vi "Begin.vi"(8 "error in":errorcluster) -> (0 "error out":errorcluster)   [LabVIEW 2015]
doc: "Called before other user functions, this VI is expected to open initial I/O refnums, load in file data, and do all program initialization. Notice that the <B>error out</B> terminal is simply used for data flow. Wiring it to other structures or subVIs ensures that this VI runs first."
uses:
  <vilib>/Rock Robotics/WPI/DriverStation/WPI_DriverStationRobotMode2.ctl
  <vilib>/Rock Robotics/WPI/Joystick/WPI_JoystickDeviceEnum.ctl
  <vilib>/Rock Robotics/WPI/Solenoid/WPI_SolenoidChannel.ctl
  <vilib>/Rock Robotics/SystemInterfaces/DIO/FPGA_DIOPWMChannel.ctl
  <vilib>/Rock Robotics/SystemInterfaces/AI/FPGA_AIChannel.ctl
  <vilib>/Rock Robotics/WPI/SafetyOutput/WPI_SafetyOutputConfigMenu.ctl
  <vilib>/Rock Robotics/SystemInterfaces/DIO/FPGA_DIOChannel.ctl
  <vilib>/Rock Robotics/WPI/Encoder/WPI_EncoderType.ctl
  <vilib>/Rock Robotics/WPI/CAN/TalonSRX/WPI_CANTalonSRX_APIFeedbackSelect.ctl
  <vilib>/Rock Robotics/WPI/CAN/TalonSRX/WPI_CANTalonSRX_APIControlMode.ctl
  <vilib>/Rock Robotics/SystemInterfaces/DIO/FPGA_DIORelayChannel.ctl
  <vilib>/Rock Robotics/SystemInterfaces/spilib/spi_bus.ctl
  Robot Global Data.vi
  <vilib>/Rock Robotics/Network Tables/NT Write String Array.vi
  <vilib>/Rock Robotics/WPI/Solenoid/WPI_SolenoidOpenSingle.vi
  <vilib>/Rock Robotics/WPI/Solenoid/Deprecated/WPI_SolenoidSetBool.vi
  <vilib>/Rock Robotics/WPI/MotorControl/WPI_MotorControlOpen Talon.vi
  <vilib>/Rock Robotics/WPI/RobotDrive/WPI_RobotDriveOpen2MotorWithVictorSP.vi
  <vilib>/Rock Robotics/WPI/Counter/WPI_CounterDigitalInputToDigitalSource.vi
  <vilib>/Rock Robotics/WPI/MotorControl/WPI_MotorControlOpenCANTalonSRX.vi
  <vilib>/Rock Robotics/WPI/MotorControl/WPI_MotorControlOpen VictorSP.vi
  <vilib>/Rock Robotics/WPI/Gyro/WPI_GyroXRS450_SPI_Open.vi
  <vilib>/Rock Robotics/WPI/Switch/WPI_SwitchOpenLimit.vi
  <vilib>/Rock Robotics/WPI/RobotDrive/WPI_RobotDriveOpen4MotorWithVictorSP.vi
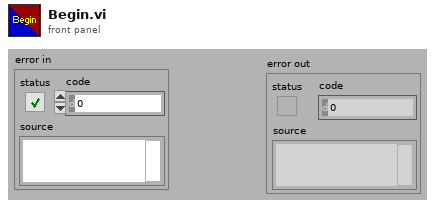
[diagram p1: front panel]
types:
  T1 = typedef "WPI_SolenoidChannel.ctl" = enum8{"Solenoid 0", "Solenoid 1", "Solenoid 2", "Solenoid 3", "Solenoid 4", "Solenoid 5", "Solenoid 6", "Solenoid 7", "Invalid"}
  T2 = typedef "FPGA_DIOPWMChannel.ctl" = enum8{"PWM 0", "PWM 1", "PWM 2", "PWM 3", "PWM 4", "PWM 5", "PWM 6", "PWM 7", "PWM 8", "PWM 9", "PWM MXP 0", "PWM MXP 1", "PWM MXP 2", "PWM MXP 3", "PWM MXP 4", "PWM MXP 5", "PWM MXP 6", "PWM MXP 7", "PWM MXP 8", "PWM MXP 9", "Invalid"}
  T3 = typedef "FPGA_DIOChannel.ctl" = enum8{"DIO 0", "DIO 1", "DIO 2", "DIO 3", "DIO 4", "DIO 5", "DIO 6", "DIO 7", "DIO 8", "DIO 9", "DIO MXP 0", "DIO MXP 1", "DIO MXP 2", "DIO MXP 3", "DIO MXP 4", "DIO MXP 5", "DIO MXP 6", "DIO MXP 7", "DIO MXP 8", "DIO MXP 9", "DIO MXP 10", "DIO MXP 11", "DIO MXP 12", "DIO MXP 13", "DIO MXP 14", "DIO MXP 15", "Invalid"}
  T4 = typedef "spi_bus.ctl" = enum16{"SPI On-Board, CS0", "SPI On-Board, CS1", "SPI On-Board, CS2", "SPI On-Board, CS3", "SPI MXP", "Invalid"}
  T5 = typedef "FPGA_AIChannel.ctl" = enum8{"AI 0", "AI 1", "AI 2", "AI 3", "AI MXP 0", "AI MXP 1", "AI MXP 2", "AI MXP 3", "Invalid"}
  T6 = typedef "FPGA_DIORelayChannel.ctl" = enum8{"Relay 0", "Relay 1", "Relay 2", "Relay 3", "Invalid"}
  T7 = typedef "WPI_CANTalonSRX_APIControlMode.ctl" = enum8{"Percent VBus", "Speed", "Position", "Slave", "Unchanged / Invalid", "Voltage Compensation", "Current", "Motion Profile"}
  T8 = typedef "WPI_CANTalonSRX_APIFeedbackSelect.ctl" = enum16{"Digital Quadrature Encoder", "Analog Potentiometer", "Analog Encoder", "Count on Quad-A (Rising-Edge)", "Count on Quad-A (Falling-Edge)", "CTR Magnetic Enc (Absolute)", "CTR Magnetic Enc (Relative)", "Pulse Width"}
  T9 = typedef "WPI_EncoderType.ctl" = enum16{"1x", "2x", "4x"}
  T10 = typedef "WPI_SafetyOutputConfigMenu.ctl" = enum16{"Enable", "Disable"}
  T11 = enum16{"Intake", "Fender", "D4", "Low Bar", "Backwards Fender"}
  T12 = typedef "WPI_JoystickDeviceEnum.ctl" = enum16{"USB 0", "USB 1", "USB 2", "USB 3", "USB 4", "USB 5"}
  T13 = typedef "WPI_DriverStationRobotMode2.ctl" = enum16{"Autonomous Disabled", "Autonomous Enabled", "Teleop Disabled", "Teleop Enabled", "Disconnected", "Finish", "Test Disabled", "Test Enabled", "Emergency Stopped"}
  T14 = typedef "WPI_MotorControlDeviceRef.ctl" = cluster{"DeviceStatus":errorcluster, "Type":T15, "PWM":cluster{"PWM Channel":T2, "DeadBand":T16}, "CAN":cluster{"Device Number":u8, "Control Mode":T17, "Semaphore":T18, "Max Vout":dbl, "TalonSRX Control Mode":T7}, "Invert":bool}
  T15 = typedef "WPI_MotorControlType.ctl" = enum16{"PWM", "CAN", "CANTalonSRX"}
  T16 = typedef "WPI_PWMDeadband.ctl" = cluster{"Name":string, "maxPositivePwm":i32, "minPositivePwm":i32, "centerPwm":i32, "maxNegativePwm":i32, "minNegativePwm":i32, "angularRange":u16}
  T17 = typedef "WPI_CANJaguar_ControlMode.ctl" = enum8{"Percent VBus", "Current", "Speed", "Position", "Voltage"}
  T18 = typedef "Semaphore RefNum" = refnum<k1>
  T19 = typedef "WPI_RobotDriveDevRef.ctl" = cluster{"DevStatus":errorcluster, "Motors[]":T14[], "Square Inputs":bool, "Max Output":dbl}
  T20 = typedef "WPI_RelayDevRef.ctl" = cluster{"DevStatus":errorcluster, "Relay Channel":T6, "Relay Direction":T21}
  T21 = typedef "WPI_RelayDirection.ctl" = enum16{"Both directions", "Forward only", "Reverse only"}
  T22 = typedef "WPI_SolenoidDevRef.ctl" = cluster{"DevStatus":errorcluster, "Pneumatics Control Module":u8, "Forward Solenoid Channel":T1, "Reverse Solenoid Channel":T1}
  T23 = typedef "WPI_GyroDevRef.ctl" = cluster{"DevStatus":errorcluster, "Analog Channel":T5, "Offset":dbl, "Gain (VoltsPerDegree/Second)":dbl, "Gyro Type":enum16{"Analog", "XRS450"}, "Handle":i32, "SPI Bus":T4, "Device Found":bool, "Sample Rate":dbl, "Calibrate On Open":bool}
  T24 = typedef "WPI_PotentiometerDevRef.ctl" = cluster{"DevStatus":errorcluster, "Analog Channel":T5, "Invert Output":bool}
  T25 = typedef "WPI_JoystickDevRef.ctl" = cluster{"Device":T12}
  T26 = typedef "WPI_SwitchDevRef.ctl" = cluster{"DevStatus":errorcluster, "DIO Channel":T3, "CntIndex":T27, "Normally Closed":bool}
  T27 = typedef "FPGA_CounterCtrSystemIndex.ctl" = enum8{"Ctr 0", "Ctr 1", "Ctr 2", "Ctr 3", "Ctr 4", "Ctr 5", "Ctr 6", "Ctr 7", "Invalid"}
  T28 = typedef "WPI_DigitalInputDevRef.ctl" = cluster{"DevStatus":errorcluster, "DIO Channel":T3}
  T29 = typedef "FPGA_CounterEncoderSourceConvertionLVSourceType.ctl" = cluster{"DevStatus":errorcluster, "AnalogTriggerMode?":bool, "DigitalMode":cluster{"DIO Channel":T30}, "AnalogTriggerMode":cluster{"AnalogTriggerIndex":T31, "OutputType":T32}}
  T30 = typedef "FPGA_DIODigitalSourceChannel.ctl" = enum8{"DIO 0", "DIO 1", "DIO 2", "DIO 3", "DIO 4", "DIO 5", "DIO 6", "DIO 7", "DIO 8", "DIO 9", "DIO MXP 0", "DIO MXP 1", "DIO MXP 2", "DIO MXP 3", "DIO MXP 4", "DIO MXP 5", "DIO MXP 6", "DIO MXP 7", "DIO MXP 8", "DIO MXP 9", "DIO MXP 10", "DIO MXP 11", "DIO MXP 12", "DIO MXP 13", "DIO MXP 14", "DIO MXP 15", "Disabled"}
  T31 = typedef "FPGA_AnalogTriggerIndex.ctl" = enum8{"Trig 0", "Trig 1", "Trig 2", "Trig 3", "Trig 4", "Trig 5", "Trig 6", "Trig 7", "Invalid"}
  T32 = typedef "FPGA_AnalogTriggerOutType.ctl" = enum16{"InWindow", "TriggerState", "Rising", "Falling"}
  T33 = typedef "WPI_AnalogChannelDevRef.ctl" = cluster{"DevStatus":errorcluster, "Analog Channel":T5}
  T34 = typedef "WPI_EncoderDevRef.ctl" = cluster{"DevStatus":errorcluster, "EncoderIndex":T35, "CounterIndex":T27, "DistancePerCount":dbl, "Decoding Type":T9}
  T35 = typedef "FPGA_EncoderIdx.ctl" = enum8{"Enc 0", "Enc 1", "Enc 2", "Enc 3", "Enc 4", "Enc 5", "Enc 6", "Enc 7", "Invalid"}
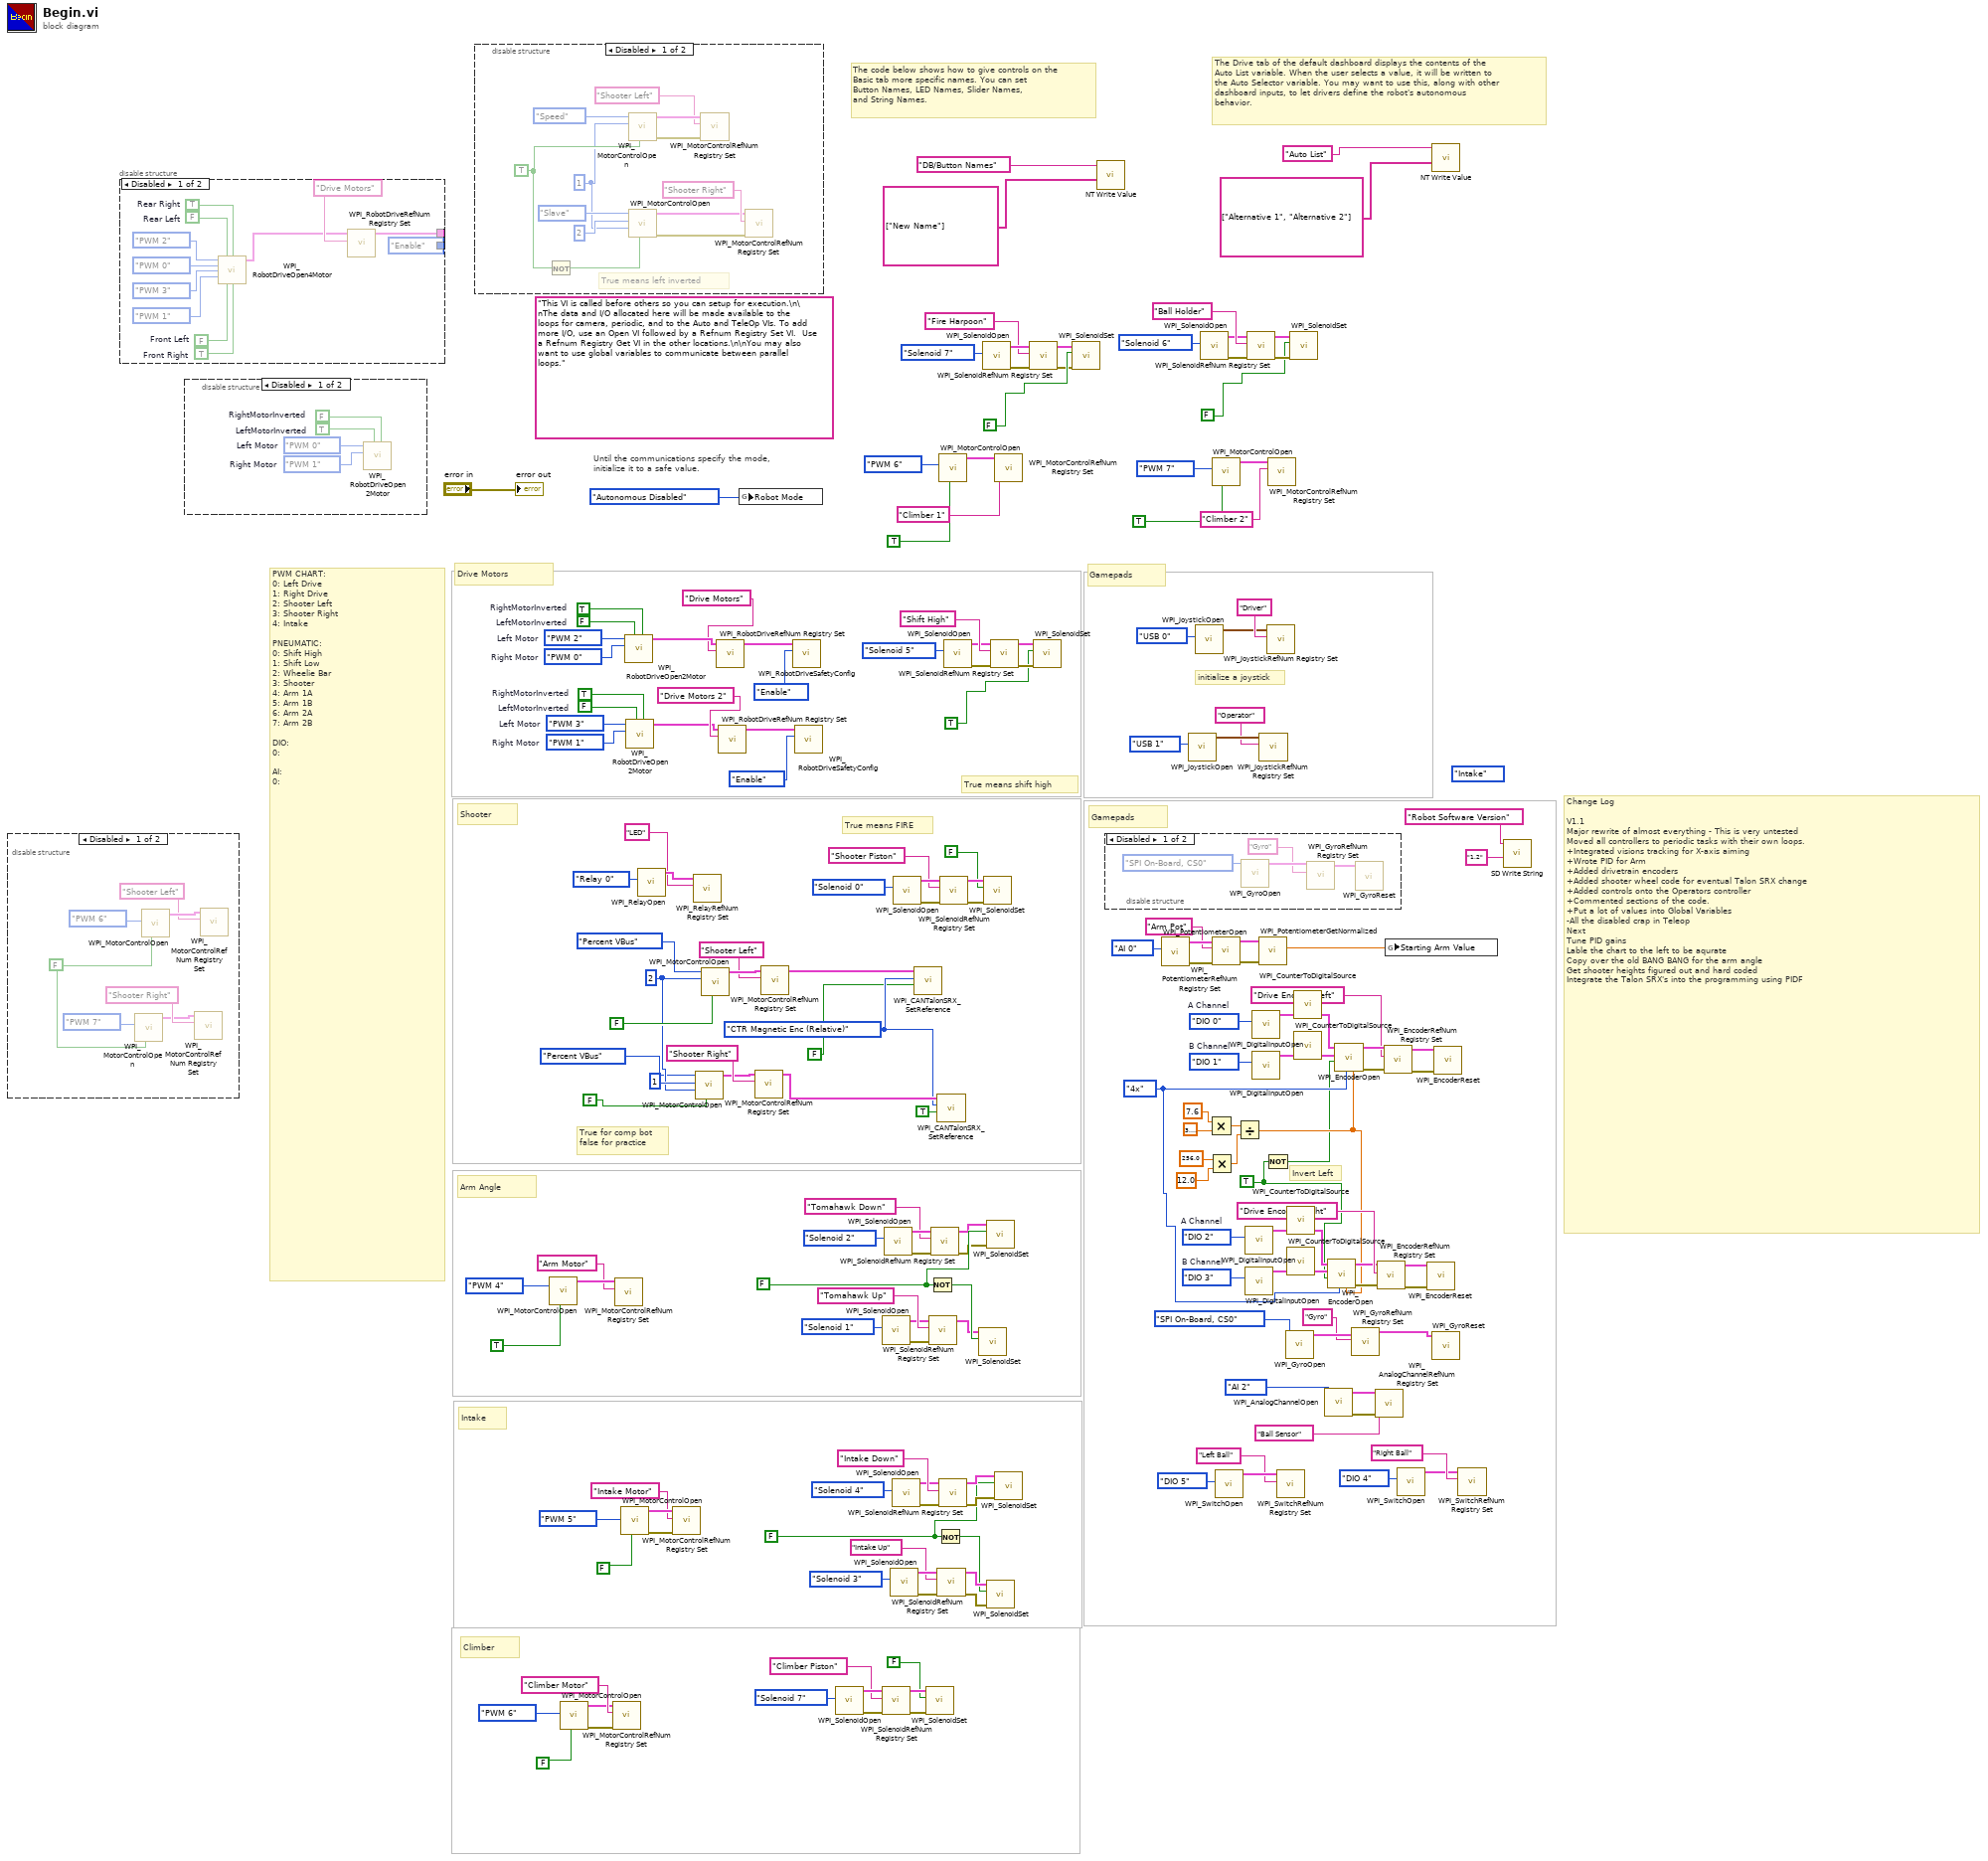
[diagram p0: block diagram]
diagram:
  w70 = FALSE
  w53 = WPI_CANTalonSRX_APIFeedbackSelect."CTR Magnetic Enc (Relative)" ("Feedback Reference")
  w75 = u8 2 ("Device Number")
  w84 = TRUE
  w88 = FPGA_DIOChannel."DIO 3"  # B Channel
  w89 = FPGA_DIOChannel."DIO 2"  # A Channel
  w87 = WPI_EncoderType."4x" ("Decoding Type")
  w114 = FPGA_DIOChannel."DIO 1"  # B Channel
  w113 = FPGA_DIOChannel."DIO 0"  # A Channel
  w117 = FPGA_DIOPWMChannel."PWM 1"  # Right Motor
  w118 = FPGA_DIOPWMChannel."PWM 3"  # Left Motor
  w119 = FALSE  # LeftMotorInverted
  w120 = TRUE  # RightMotorInverted
  w132 = FPGA_DIOPWMChannel."PWM 0"  # Right Motor
  w131 = FPGA_DIOPWMChannel."PWM 2"  # Left Motor
  w130 = FALSE  # LeftMotorInverted
  w129 = TRUE  # RightMotorInverted
  (unwired) T11."Intake"
  w153 = FALSE
  (unwired) "This VI is called before others so you can setup for execution.\n\nThe data and I/O allocated here will be made available to the loops for camera, periodic, and to the Auto and TeleOp VIs. To add more I/O, use an Open VI followed by a Refnum Registry Set VI.  Use a Refnum Registry Get VI in the other locations.\n\nYou may also want to use global variables to communicate between parallel loops."
  # "Climber"
  # "True for comp bot\nfalse for practice"
  # "Change Log\n \nV1.1\nMajor rewrite of almost everything - This is very untested\nMoved all controllers to periodic tasks with their own loops.\n+Integrated visions tracking for X-axis aiming\n+Wrote PID for Arm\n+Added drivetrain encoders\n+Added shooter wheel code for eventual Talon SRX change\n+Added controls onto the Operators controller \n+Commented sections of the code.\n+Put a lot of values into Global Variables\n-All the disabled crap in Teleop\nNext\nTune PID gains\nLable the chart to the left to be aqurate\nCopy over the old BANG BANG for the arm angle\nGet shooter heights figured out and hard coded\nIntegrate the Talon SRX's into the programming using PIDF"
  # "Invert Left"
  # "Gamepads"
  # "True means FIRE"
  # "True means shift high"
  # "Intake"
  # "Arm Angle"
  # "Shooter"
  # "Gamepads"
  # "Drive Motors"
  # "PWM CHART:\n0: Left Drive\n1: Right Drive\n2: Shooter Left\n3: Shooter Right\n4: Intake \n\nPNEUMATIC:\n0: Shift High\n1: Shift Low\n2: Wheelie Bar\n3: Shooter \n4: Arm 1A\n5: Arm 1B\n6: Arm 2A\n7: Arm 2B \n\nDIO:\n0: \n\nAI:\n0:"
  # "The Drive tab of the default dashboard displays the contents of the\nAuto List variable. When the user selects a value, it will be written to\nthe Auto Selector variable. You may want to use this, along with other\ndashboard inputs, to let drivers define the robot's autonomous\nbehavior."
  # "The code below shows how to give controls on the\nBasic tab more specific names. You can set\nButton Names, LED Names, Slider Names,\nand String Names."
  # "initialize a joystick"
  # "Until the communications specify the mode,\ninitialize it to a safe value."
  n1 = disable-structure shown="Disabled" {
    frame Disabled {
      w186 = FALSE
      n2 = call-poly <vilib>:"WPI_MotorControlOpen.vi"("Invert"=w186, "PWM Channel"=FPGA_DIOPWMChannel."PWM 7") -> ("MotorControlDeviceRef"=w188:T14)  [unwired: 8 in, 1 out]
      n3 = call-poly <vilib>:"WPI_MotorControlOpen.vi"("Invert"=w186, "PWM Channel"=FPGA_DIOPWMChannel."PWM 6") -> ("MotorControlDeviceRef"=w191:T14)  [unwired: 8 in, 1 out]
      n4 = call <vilib>:"WPI_MotorControlRefNum Registry Set.vi"("refnum name"="Shooter Right", "MotorControlDevRef"=w188) -> ()  [unwired: 8 in, 2 out]
      n5 = call <vilib>:"WPI_MotorControlRefNum Registry Set.vi"("refnum name"="Shooter Left", "MotorControlDevRef"=w191) -> ()  [unwired: 8 in, 2 out]
    }
    frame Enabled {
    }
  }
  n6 = disable-structure shown="Disabled" {
    disable-tunnel: [w203 _] -> _
    disable-tunnel: [WPI_SafetyOutputConfigMenu."Enable" ("mode") _] -> _
    frame Disabled {
      w195 = FALSE  # Rear Left
      w194 = TRUE  # Rear Right
      w196 = TRUE  # Front Right
      w197 = FALSE  # Front Left
      n7 = call-poly <vilib>:"WPI_RobotDriveOpen4Motor.vi"("Rear Left Motor"=FPGA_DIOPWMChannel."PWM 2", "Rear Left Motor Inverted"=w195, "Rear Right Motor Inverted"=w194, "Rear Right Motor"=FPGA_DIOPWMChannel."PWM 0", "Front Left Motor"=FPGA_DIOPWMChannel."PWM 3", "Front Right Motor"=FPGA_DIOPWMChannel."PWM 1", "Front Left Motor Inverted"=w197, "Front Right Motor Inverted"=w196) -> ("RobotDriveDevRef"=w193:T19)  [unwired: 6 in, 1 out]
      n8 = call <vilib>:"WPI_RobotDriveRefNum Registry Set.vi"("refnum name"="Drive Motors", "RobotDriveDevRef"=w193) -> ("RobotDriveDevRef"=w203:T19)  [unwired: 2 in, 7 out]
    }
    frame Enabled {
    }
  }
  n9 = disable-structure shown="Disabled" {
    frame Disabled {
      w205 = FPGA_DIOPWMChannel."PWM 1"  # Right Motor
      w206 = FPGA_DIOPWMChannel."PWM 0"  # Left Motor
      w207 = TRUE  # LeftMotorInverted
      w208 = FALSE  # RightMotorInverted
      n10 = call-poly <vilib>:"WPI_RobotDriveOpen2Motor.vi"("Right Motor Inverted"=w208, "Left Motor Inverted"=w207, "Right Motor"=w205, "Left Motor"=w206) -> ()  [unwired: 1 in, 7 out]
    }
    frame Enabled {
    }
  }
  n11 = disable-structure shown="Disabled" {
    frame Disabled {
      w209 = u8 1 ("Device Number")
      w213 = TRUE
      # "True means left inverted"
      n12 = Not(x=w213) -> (.not. x?=w214:bool)
      n13 = call-poly <vilib>:"WPI_MotorControlOpen.vi"("Invert"=w213, "Device Number"=w209, "Control Mode"=WPI_CANTalonSRX_APIControlMode."Speed") -> ("error out"=w220:errorcluster, "MotorControlDeviceRef"=w219:T14)  [unwired: 7 in]
      n14 = call-poly <vilib>:"WPI_MotorControlOpen.vi"("Invert"=w214, "Master Device Number"=w209, "Device Number"=u8 2, "Control Mode"=WPI_CANTalonSRX_APIControlMode."Slave") -> ("error out"=w215:errorcluster, "MotorControlDeviceRef"=w216:T14)  [unwired: 6 in]
      n15 = call <vilib>:"WPI_MotorControlRefNum Registry Set.vi"("error in (no error)"=w220, "refnum name"="Shooter Left", "MotorControlDevRef"=w219) -> ()  [unwired: 7 in, 2 out]
      n16 = call <vilib>:"WPI_MotorControlRefNum Registry Set.vi"("error in (no error)"=w215, "refnum name"="Shooter Right", "MotorControlDevRef"=w216) -> ()  [unwired: 7 in, 2 out]
    }
    frame Enabled {
    }
  }
  n17 = call-poly <vilib>:"WPI_MotorControlOpen.vi"("Invert"=TRUE, "PWM Channel"=FPGA_DIOPWMChannel."PWM 4") -> ("MotorControlDeviceRef"=w141:T14)  [unwired: 8 in, 1 out]
  n18 = call-poly <vilib>:"WPI_MotorControlOpen.vi"("Invert"=FALSE, "PWM Channel"=FPGA_DIOPWMChannel."PWM 6") -> ("error out"=w8:errorcluster, "MotorControlDeviceRef"=w9:T14)  [unwired: 8 in]
  n19 = call <vilib>:"WPI_MotorControlRefNum Registry Set.vi"("error in (no error)"=w8, "refnum name"="Climber Motor", "MotorControlDevRef"=w9) -> ()  [unwired: 7 in, 2 out]
  n20 = call <vilib>:"WPI_MotorControlRefNum Registry Set.vi"("refnum name"="Arm Motor", "MotorControlDevRef"=w141) -> ()  [unwired: 8 in, 2 out]
  n21 = call-poly <vilib>:"WPI_MotorControlOpen.vi"("Invert"=FALSE, "PWM Channel"=FPGA_DIOPWMChannel."PWM 5") -> ("error out"=w152:errorcluster, "MotorControlDeviceRef"=w151:T14)  [unwired: 8 in]
  n22 = call-poly <vilib>:"WPI_RobotDriveOpen2Motor.vi"("Right Motor Inverted"=w129, "Left Motor Inverted"=w130, "Right Motor"=w132, "Left Motor"=w131) -> ("RobotDriveDevRef"=w128:T19)  [unwired: 1 in, 6 out]
  n23 = call-poly <vilib>:"WPI_RobotDriveOpen2Motor.vi"("Right Motor Inverted"=w120, "Left Motor Inverted"=w119, "Right Motor"=w117, "Left Motor"=w118) -> ("RobotDriveDevRef"=w121:T19)  [unwired: 1 in, 6 out]
  n24 = call <vilib>:"WPI_RelayOpen.vi"("Relay Channel"=FPGA_DIORelayChannel."Relay 0") -> ("RelayDevRef"=w57:T20)  [unwired: 9 in, 1 out]
  n25 = call <vilib>:"WPI_MotorControlRefNum Registry Set.vi"("error in (no error)"=w152, "refnum name"="Intake Motor", "MotorControlDevRef"=w151) -> ()  [unwired: 7 in, 2 out]
  n26 = call <vilib>:"WPI_RelayRefNum Registry Set.vi"("refnum name"="LED", "RelayDevRef"=w57) -> ()  [unwired: 8 in, 2 out]
  n27 = call-poly <vilib>:"WPI_MotorControlOpen.vi"("Invert"=FALSE, "Master Device Number"=w75, "Device Number"=u8 1, "Control Mode"=WPI_CANTalonSRX_APIControlMode."Percent VBus") -> ("MotorControlDeviceRef"=w78:T14)  [unwired: 6 in, 1 out]
  n28 = call-poly <vilib>:"WPI_MotorControlOpen.vi"("Invert"=FALSE, "Device Number"=w75, "Control Mode"=WPI_CANTalonSRX_APIControlMode."Percent VBus") -> ("MotorControlDeviceRef"=w81:T14)  [unwired: 7 in, 1 out]
  n29 = call <vilib>:"WPI_RobotDriveRefNum Registry Set.vi"("refnum name"="Drive Motors", "RobotDriveDevRef"=w128) -> ("RobotDriveDevRef"=w127:T19)  [unwired: 2 in, 7 out]
  n30 = call <vilib>:"WPI_RobotDriveRefNum Registry Set.vi"("refnum name"="Drive Motors 2", "RobotDriveDevRef"=w121) -> ("RobotDriveDevRef"=w122:T19)  [unwired: 2 in, 7 out]
  n31 = global write "Robot Global Data.vi" "Robot Mode"(WPI_DriverStationRobotMode2."Autonomous Disabled" ("Robot Mode")) -> ()
  n32 = call <vilib>:"WPI_MotorControlRefNum Registry Set.vi"("refnum name"="Shooter Right", "MotorControlDevRef"=w78) -> ("MotorControlDevRef"=w54:T14)  [unwired: 8 in, 1 out]
  n33 = call <vilib>:"WPI_MotorControlRefNum Registry Set.vi"("refnum name"="Shooter Left", "MotorControlDevRef"=w81) -> ("MotorControlDevRef"=w73:T14)  [unwired: 8 in, 1 out]
  n34 = call <vilib>:"WPI_RobotDriveSafetyConfig.vi"("mode"=WPI_SafetyOutputConfigMenu."Enable", "RobotDriveDevRef"=w127) -> ()  [unwired: 8 in, 2 out]
  n35 = call <vilib>:"WPI_RobotDriveSafetyConfig.vi"("mode"=WPI_SafetyOutputConfigMenu."Enable", "RobotDriveDevRef"=w122) -> ()  [unwired: 8 in, 2 out]
  n36 = call-poly <vilib>:"WPI_SolenoidOpen.vi"("Solenoid Channel"=WPI_SolenoidChannel."Solenoid 7") -> ("error out"=w7:errorcluster, "SolenoidDevRef"=w6:T22)  [unwired: 9 in]
  n37 = call-poly <vilib>:"WPI_SolenoidOpen.vi"("Solenoid Channel"=WPI_SolenoidChannel."Solenoid 1") -> ("error out"=w62:errorcluster, "SolenoidDevRef"=w63:T22)  [unwired: 9 in]
  n38 = call <vilib>:"WPI_SolenoidRefNum Registry Set.vi"("error in (no error)"=w7, "refnum name"="Climber Piston", "SolenoidDevRef"=w6) -> ("error out"=w3:errorcluster, "SolenoidDevRef"=w2:T22)  [unwired: 7 in]
  n39 = call-poly <vilib>:"WPI_SolenoidOpen.vi"("Solenoid Channel"=WPI_SolenoidChannel."Solenoid 2") -> ("error out"=w61:errorcluster, "SolenoidDevRef"=w60:T22)  [unwired: 9 in]
  n40 = call-poly <vilib>:"WPI_SolenoidOpen.vi"("Solenoid Channel"=WPI_SolenoidChannel."Solenoid 3") -> ("error out"=w162:errorcluster, "SolenoidDevRef"=w161:T22)  [unwired: 9 in]
  n41 = call-poly <vilib>:"WPI_SolenoidOpen.vi"("Solenoid Channel"=WPI_SolenoidChannel."Solenoid 4") -> ("error out"=w163:errorcluster, "SolenoidDevRef"=w164:T22)  [unwired: 9 in]
  n42 = call-poly <vilib>:"WPI_SolenoidOpen.vi"("Solenoid Channel"=WPI_SolenoidChannel."Solenoid 0") -> ("error out"=w173:errorcluster, "SolenoidDevRef"=w172:T22)  [unwired: 9 in]
  n43 = call <vilib>:"WPI_CANTalonSRX_SetReference.vi"("Reverse Feedback Sensor"=FALSE, "Feedback Reference"=w53, "CAN Talon SRX Ref"=w73) -> ()  [unwired: 7 in, 2 out]
  n44 = call-poly <vilib>:"WPI_SolenoidSet.vi"("error in (no error)"=w3, "Value"=FALSE, "SolenoidDevRef"=w2) -> ()  [unwired: 7 in, 2 out]
  n45 = Not(x=w70) -> (.not. x?=w69:bool)
  n46 = call <vilib>:"WPI_SolenoidRefNum Registry Set.vi"("error in (no error)"=w62, "refnum name"="Tomahawk Up", "SolenoidDevRef"=w63) -> ("SolenoidDevRef"=w66:T22)  [unwired: 7 in, 1 out]
  n47 = call <vilib>:"WPI_SolenoidRefNum Registry Set.vi"("error in (no error)"=w61, "refnum name"="Tomahawk Down", "SolenoidDevRef"=w60) -> ("error out"=w67:errorcluster, "SolenoidDevRef"=w68:T22)  [unwired: 7 in]
  n48 = Not(x=w153) -> (.not. x?=w154:bool)
  n49 = call <vilib>:"WPI_CANTalonSRX_SetReference.vi"("Reverse Feedback Sensor"=TRUE, "Feedback Reference"=w53, "CAN Talon SRX Ref"=w54) -> ()  [unwired: 7 in, 2 out]
  n50 = call <vilib>:"WPI_SolenoidRefNum Registry Set.vi"("error in (no error)"=w162, "refnum name"="Intake Up", "SolenoidDevRef"=w161) -> ("error out"=w158:errorcluster, "SolenoidDevRef"=w157:T22)  [unwired: 7 in]
  n51 = call-poly <vilib>:"WPI_MotorControlOpen.vi"("Invert"=TRUE, "PWM Channel"=FPGA_DIOPWMChannel."PWM 6") -> ("MotorControlDeviceRef"=w28:T14)  [unwired: 8 in, 1 out]
  n52 = call <vilib>:"WPI_SolenoidRefNum Registry Set.vi"("error in (no error)"=w163, "refnum name"="Intake Down", "SolenoidDevRef"=w164) -> ("error out"=w156:errorcluster, "SolenoidDevRef"=w155:T22)  [unwired: 7 in]
  n53 = call <vilib>:"WPI_SolenoidRefNum Registry Set.vi"("error in (no error)"=w173, "refnum name"="Shooter Piston", "SolenoidDevRef"=w172) -> ("error out"=w169:errorcluster, "SolenoidDevRef"=w168:T22)  [unwired: 7 in]
  n54 = call-poly <vilib>:"WPI_SolenoidOpen.vi"("Solenoid Channel"=WPI_SolenoidChannel."Solenoid 5") -> ("error out"=w144:errorcluster, "SolenoidDevRef"=w145:T22)  [unwired: 9 in]
  n55 = call-poly <vilib>:"WPI_SolenoidSet.vi"("Value"=w69, "SolenoidDevRef"=w66) -> ()  [unwired: 8 in, 2 out]
  n56 = call-poly <vilib>:"WPI_SolenoidOpen.vi"("Solenoid Channel"=WPI_SolenoidChannel."Solenoid 7") -> ("error out"=w39:errorcluster, "SolenoidDevRef"=w38:T22)  [unwired: 9 in]
  n57 = call-poly <vilib>:"WPI_SolenoidSet.vi"("error in (no error)"=w169, "Value"=FALSE, "SolenoidDevRef"=w168) -> ()  [unwired: 7 in, 2 out]
  n58 = call-poly <vilib>:"WPI_SolenoidSet.vi"("error in (no error)"=w67, "Value"=w70, "SolenoidDevRef"=w68) -> ()  [unwired: 7 in, 2 out]
  n59 = call-poly <vilib>:"WPI_SolenoidSet.vi"("error in (no error)"=w158, "Value"=w154, "SolenoidDevRef"=w157) -> ()  [unwired: 7 in, 2 out]
  n60 = call <vilib>:"WPI_SolenoidRefNum Registry Set.vi"("error in (no error)"=w144, "refnum name"="Shift High", "SolenoidDevRef"=w145) -> ("error out"=w143:errorcluster, "SolenoidDevRef"=w142:T22)  [unwired: 7 in]
  n61 = call <vilib>:"WPI_MotorControlRefNum Registry Set.vi"("refnum name"="Climber 1", "MotorControlDevRef"=w28) -> ()  [unwired: 8 in, 2 out]
  n62 = call-poly <vilib>:"WPI_SolenoidSet.vi"("error in (no error)"=w156, "Value"=w153, "SolenoidDevRef"=w155) -> ()  [unwired: 7 in, 2 out]
  n63 = call <vilib>:"WPI_SolenoidRefNum Registry Set.vi"("error in (no error)"=w39, "refnum name"="Fire Harpoon", "SolenoidDevRef"=w38) -> ("error out"=w40:errorcluster, "SolenoidDevRef"=w41:T22)  [unwired: 7 in]
  n64 = call-poly <vilib>:"WPI_SolenoidSet.vi"("error in (no error)"=w143, "Value"=TRUE, "SolenoidDevRef"=w142) -> ()  [unwired: 7 in, 2 out]
  n65 = call-poly <vilib>:"WPI_SolenoidSet.vi"("error in (no error)"=w40, "Value"=FALSE, "SolenoidDevRef"=w41) -> ()  [unwired: 7 in, 2 out]
  n66 = call-poly <vilib>:"NT Write Value.vi"("String Array"=string[] ["New Name"], "Name"="DB/Button Names") -> ()  [unwired: 9 in, 1 out]
  n67 = disable-structure shown="Disabled" {
    frame Disabled {
      n68 = call-poly <vilib>:"WPI_GyroOpen.vi"("SPI Bus"=spi_bus."SPI On-Board, CS0") -> ("GyroDevRef"=w224:T23)  [unwired: 9 in, 1 out]
      n69 = call <vilib>:"WPI_GyroRefNum Registry Set.vi"("refnum name"="Gyro", "GyroDevRef"=w224) -> ("GyroDevRef"=w223:T23)  [unwired: 8 in, 1 out]
      n70 = call <vilib>:"WPI_GyroReset.vi"("GyroDevRef"=w223) -> ()  [unwired: 9 in, 2 out]
    }
    frame Enabled {
    }
  }
  n71 = call <vilib>:"WPI_PotentiometerOpen.vi"("Analog Channel"=FPGA_AIChannel."AI 0") -> ("error out"=w139:errorcluster, "PotDevRef"=w138:T24)  [unwired: 9 in]
  n72 = call <vilib>:"WPI_JoystickOpen.vi"("JoystickDevice"=WPI_JoystickDeviceEnum."USB 1") -> ("JoystickDevRef"=w175:T25)  [unwired: 10 in]
  n73 = call <vilib>:"WPI_JoystickOpen.vi"("JoystickDevice"=WPI_JoystickDeviceEnum."USB 0") -> ("JoystickDevRef"=w183:T25)  [unwired: 10 in]
  n74 = call-poly <vilib>:"WPI_SolenoidOpen.vi"("Solenoid Channel"=WPI_SolenoidChannel."Solenoid 6") -> ("error out"=w32:errorcluster, "SolenoidDevRef"=w33:T22)  [unwired: 9 in]
  n75 = Multiply(x=7.6, y=3.141592653589793) -> (x*y=w99:dbl)
  n76 = Multiply(x=256.0, y=12.0) -> (x*y=w102:dbl)
  n77 = call-poly <vilib>:"WPI_MotorControlOpen.vi"("Invert"=TRUE, "PWM Channel"=FPGA_DIOPWMChannel."PWM 7") -> ("MotorControlDeviceRef"=w25:T14)  [unwired: 8 in, 1 out]
  n78 = call <vilib>:"WPI_PotentiometerRefNum Registry Set.vi"("error in (no error)"=w139, "refnum name"="Arm Pot", "PotDevRef"=w138) -> ("error out"=w135:errorcluster, "PotDevRef"=w134:T24)  [unwired: 7 in]
  n79 = call-poly <vilib>:"WPI_SwitchOpen.vi"("DIO Channel"=FPGA_DIOChannel."DIO 5") -> ("SwitchDevRef"=w19:T26)  [unwired: 9 in, 1 out]
  n80 = Divide(x=w99, y=w102) -> (x/y=w86:dbl)
  n81 = call <vilib>:"WPI_DigitalInputOpen.vi"("DIO Channel"=w89) -> ("DigitalInputDevRef"=w92:T28)  [unwired: 1 in, 9 out]
  n82 = call <vilib>:"WPI_DigitalInputOpen.vi"("DIO Channel"=w88) -> ("DigitalInputDevRef"=w91:T28)  [unwired: 1 in, 9 out]
  n83 = call <vilib>:"WPI_SolenoidRefNum Registry Set.vi"("error in (no error)"=w32, "refnum name"="Ball Holder", "SolenoidDevRef"=w33) -> ("error out"=w31:errorcluster, "SolenoidDevRef"=w30:T22)  [unwired: 7 in]
  n84 = call <vilib>:"WPI_DigitalInputOpen.vi"("DIO Channel"=w113) -> ("DigitalInputDevRef"=w110:T28)  [unwired: 1 in, 9 out]
  n85 = call <vilib>:"WPI_DigitalInputOpen.vi"("DIO Channel"=w114) -> ("DigitalInputDevRef"=w111:T28)  [unwired: 1 in, 9 out]
  n86 = call <vilib>:"WPI_PotentiometerGetNormalized.vi"("error in"=w135, "PotDevRef"=w134) -> ("Normalized Value"=w133:dbl)  [unwired: 7 in, 2 out]
  n87 = call <vilib>:"WPI_JoystickRefNum Registry Set.vi"("refnum name"="Operator", "JoystickDevRef"=w175) -> ()  [unwired: 8 in, 2 out]
  n88 = Not(x=w84) -> (.not. x?=w85:bool)
  n89 = call <vilib>:"WPI_JoystickRefNum Registry Set.vi"("refnum name"="Driver", "JoystickDevRef"=w183) -> ()  [unwired: 8 in, 2 out]
  n90 = call <vilib>:"WPI_MotorControlRefNum Registry Set.vi"("refnum name"="Climber 2", "MotorControlDevRef"=w25) -> ()  [unwired: 8 in, 2 out]
  n91 = call <vilib>:"WPI_SwitchRefNum Registry Set.vi"("refnum name"="Left Ball", "SwitchDevRef"=w19) -> ()  [unwired: 8 in, 2 out]
  n92 = call-poly <vilib>:"WPI_GyroOpen.vi"("SPI Bus"=spi_bus."SPI On-Board, CS0") -> ("GyroDevRef"=w50:T23)  [unwired: 9 in, 1 out]
  n93 = call-poly <vilib>:"WPI_CounterToDigitalSource.vi"("DigitalInputDevRef"=w92) -> ("Digital Source"=w93:T29)  [unwired: 6 out]
  n94 = call-poly <vilib>:"WPI_CounterToDigitalSource.vi"("DigitalInputDevRef"=w91) -> ("Digital Source"=w90:T29)  [unwired: 6 out]
  n95 = call-poly <vilib>:"WPI_SolenoidSet.vi"("error in (no error)"=w31, "Value"=FALSE, "SolenoidDevRef"=w30) -> ()  [unwired: 7 in, 2 out]
  n96 = call-poly <vilib>:"WPI_CounterToDigitalSource.vi"("DigitalInputDevRef"=w110) -> ("Digital Source"=w109:T29)  [unwired: 6 out]
  n97 = call-poly <vilib>:"WPI_CounterToDigitalSource.vi"("DigitalInputDevRef"=w111) -> ("Digital Source"=w112:T29)  [unwired: 6 out]
  n98 = call <vilib>:"WPI_AnalogChannelOpen.vi"("Analog Channel"=FPGA_AIChannel."AI 2") -> ("error out"=w46:errorcluster, "AIDeviceRef"=w45:T33)  [unwired: 9 in]
  n99 = call <vilib>:"WPI_EncoderOpen.vi"("DistancePerCount"=w86, "Decoding Type"=w87, "Invert Direction (False)"=w84, "BSource"=w90, "ASource"=w93) -> ("error out"=w94:errorcluster, "EncoderDevRef"=w95:T34)  [unwired: 3 in, 2 out]
  n100 = call <vilib>:"WPI_EncoderOpen.vi"("DistancePerCount"=w86, "Decoding Type"=w87, "Invert Direction (False)"=w85, "BSource"=w112, "ASource"=w109) -> ("error out"=w108:errorcluster, "EncoderDevRef"=w107:T34)  [unwired: 3 in, 2 out]
  n101 = call <vilib>:"WPI_GyroRefNum Registry Set.vi"("refnum name"="Gyro", "GyroDevRef"=w50) -> ("GyroDevRef"=w49:T23)  [unwired: 8 in, 1 out]
  n102 = call <vilib>:"WPI_AnalogChannelRefNum Registry Set.vi"("error in (no error)"=w46, "refnum name"="Ball Sensor", "AIDeviceRef"=w45) -> ()  [unwired: 7 in, 2 out]
  n103 = call <vilib>:"WPI_EncoderRefNum Registry Set.vi"("error in (no error)"=w94, "refnum name"="Drive Encoder Right", "EncoderDevRef"=w95) -> ("error out"=w96:errorcluster, "EncoderDevRef"=w97:T34)  [unwired: 7 in]
  n104 = call <vilib>:"WPI_EncoderRefNum Registry Set.vi"("error in (no error)"=w108, "refnum name"="Drive Encoder Left", "EncoderDevRef"=w107) -> ("error out"=w106:errorcluster, "EncoderDevRef"=w105:T34)  [unwired: 7 in]
  n105 = global write "Robot Global Data.vi" "Starting Arm Value"(w133) -> ()
  n106 = call-poly <vilib>:"WPI_SwitchOpen.vi"("DIO Channel"=FPGA_DIOChannel."DIO 4") -> ("SwitchDevRef"=w14:T26)  [unwired: 9 in, 1 out]
  n107 = call <vilib>:"WPI_EncoderReset.vi"("error in (no error)"=w96, "EncoderDevRef"=w97) -> ()  [unwired: 8 in, 2 out]
  n108 = call-poly <vilib>:"NT Write Value.vi"("String Array"=string[] ["Alternative 1", "Alternative 2"], "Name"="Auto List") -> ()  [unwired: 9 in, 1 out]
  n109 = call <vilib>:"WPI_GyroReset.vi"("GyroDevRef"=w49) -> ()  [unwired: 9 in, 2 out]
  n110 = call <vilib>:"WPI_EncoderReset.vi"("error in (no error)"=w106, "EncoderDevRef"=w105) -> ()  [unwired: 8 in, 2 out]
  n111 = call <vilib>:"WPI_SwitchRefNum Registry Set.vi"("refnum name"="Right Ball", "SwitchDevRef"=w14) -> ()  [unwired: 8 in, 2 out]
  n112 = call <vilib>:"SD Write String.vi"("String"="1.2", "Name"="Robot Software Version") -> ()  [unwired: 8 in, 2 out]
  "error out" <- "error in"
